vi "merFISH_move_to_XY_REF_position.vi"(5 "REF #":i32, 6 "Global parameters":T1 {"# repetitions" min=0; "Dt (s)" min=0 step=1; "Filter list" items=["ET665lp", "zet405/488/561/640m", "None", "None", "None", "None"]}, 7 "XY positions":dbl[][](array[numeric]), 8 "queue ASI stage":refnum<queue>, 10 "error in":errorcluster, 11 "REF positions":dbl[][](array[numeric])) -> (0 "Global parameters out":T1 {"# repetitions" min=0; "Dt (s)" min=0 step=1; "Filter list" items=["ET665lp", "zet405/488/561/640m", "None", "None", "None", "None"]}, 1 "error out":errorcluster, 3 "XY positions":dbl[][](array[numeric]))   [LabVIEW 2015]
uses:
  CONTROLS/Global parameters.ctl
  CONTROLS/Q_ASI_stage_element.ctl
  GLOBAL/Global_ASI_stage.vi
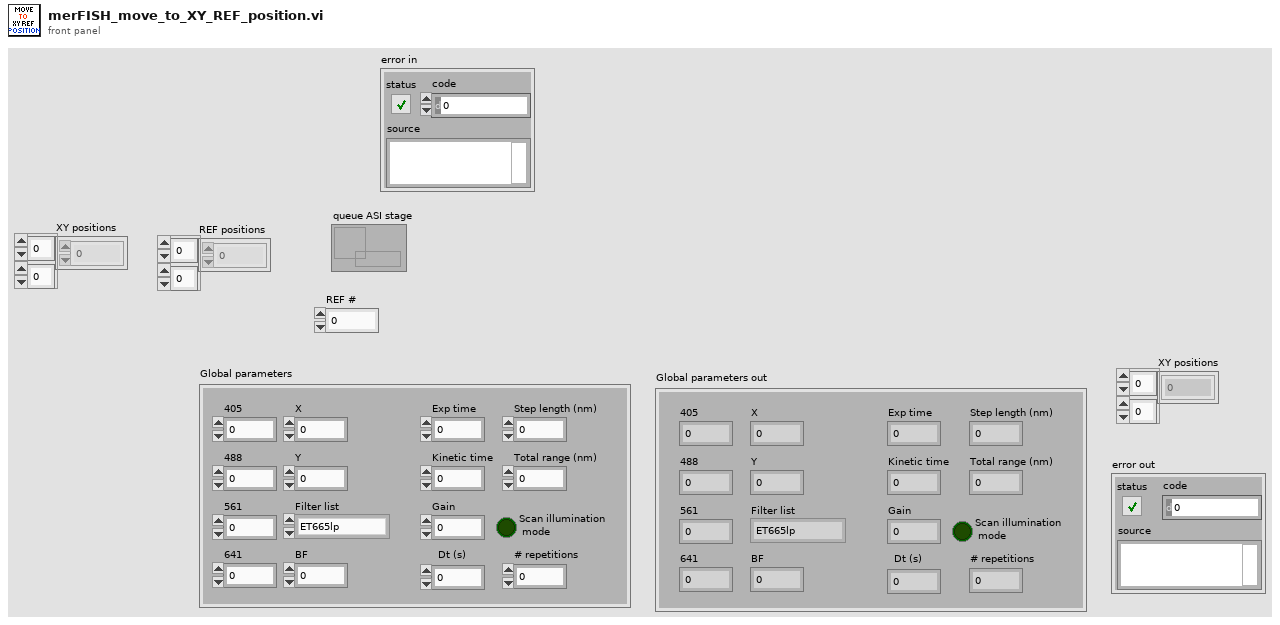
[diagram p1: front panel]
types:
  T1 = typedef "Global parameters.ctl" = cluster{"405":dbl, "488":dbl, "561":dbl, "641":dbl, "BF":dbl, "X":dbl, "Y":dbl, "Filter list":u16, "Exp time":sgl, "Kinetic time":sgl, "Gain":i32, "Step length (nm)":u32, "Total range (nm)":u32, "Scan illumination\n mode":bool, "Dt (s)":i32, "# repetitions":i32}
  T2 = typedef "Q_ASI_stage_element.ctl" = cluster{"variant":variant, "Instruction":enum16{"ASI_idle", "ASI_initialize", "ASI_error", "ASI_security_stop", "ASI_read_XYZ", "ASI_up", "ASI_down", "ASI_left", "ASI_right", "ASI_save_XY", "ASI_move_to_XY", "ASI_brightfield", "ASI_init_scan", "ASI_init_merFISH", "ASI_move_to_XY_merFISH", "ASI_move_to_Z_merFISH", "ASI_init_autofocus_search_merFISH", "ASI_close_autofocus_search_merFISH", "ASI_adjust_piezo_autofocus_merFISH", "ASI_set_piezo_autofocus_to_reference_position_merFISH_TL", "ASI_close_merFISH", "ASI_stop"}}
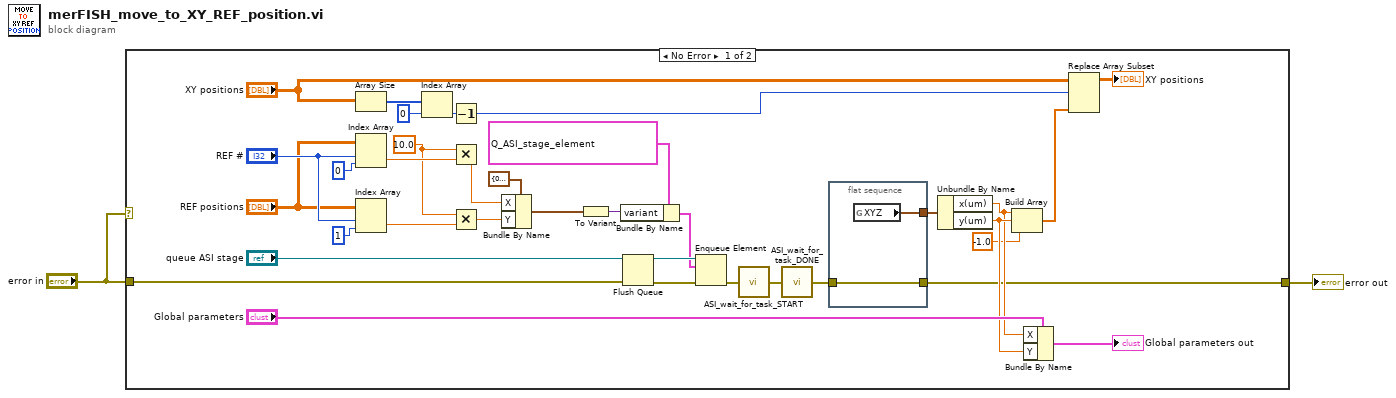
[diagram p0: block diagram]
diagram:
  n1 = case shown="No Error" "error in" {
    tunnel: "error in" -> [w26 w40]
    tunnel: [w7 w40] -> w2
    frame No Error {
      w28 = 10.0
      n2 = Array Size(array="XY positions") -> (size(s)=w36:i32[])
      n3 = Index Array(array="REF positions", index (row)="REF #", index (col)=0 ("disabled index (col)")) -> (element=w29:dbl)
      n4 = Index Array(array="REF positions", index (row)="REF #", index (col)=1 ("disabled index (col)")) -> (element=w30:dbl)
      n5 = Index Array(array=w36, index=0) -> (element=w34:i32)
      n6 = Decrement(x=w34) -> (x-1=w33:i32)
      n7 = Multiply(x=w28, y=w29) -> (x*y=w18:dbl)
      n8 = Multiply(x=w28, y=w30) -> (x*y=w17:dbl)
      n9 = Bundle By Name(cluster=cluster{"X":dbl, "Y":dbl} {"X"=0.0, "Y"=0.0} ("output cluster"), "X"=w18, "Y"=w17) -> (w5:cluster{"X":dbl, "Y":dbl})
      n10 = To Variant(anything=w5) -> (Variant=w22:variant)
      n11 = Bundle By Name(cluster=T2 {"variant"=variant, "Instruction"=enum."ASI_move_to_XY_merFISH"} ("Q_ASI_stage"), "variant"=w22) -> (w21:T2)
      n12 = Flush Queue(queue="queue ASI stage", error in (no error)=w26) -> (queue out=w24:refnum<queue>, error out=w25:errorcluster)  [unwired: 1 out]
      n13 = Enqueue Element(queue=w24, element=w21, error in (no error)=w25) -> (error out=w20:errorcluster)  [unwired: 1 in, 2 out]
      n14 = call "ASI_wait_for_task_START.vi"("error in"=w20) -> ("error out"=w19:errorcluster)
      n15 = call "ASI_wait_for_task_DONE.vi"("error in"=w19) -> ("error out"=w16:errorcluster)
      n16 = flat-sequence {
        tunnel: w16 -> [w39]
        tunnel: [w39] -> w7
        tunnel: [w38] -> w15
        frame #0 {
          n17 = global read "Global_ASI_stage.vi" "XYZ"() -> (w38:cluster{"x(um)":dbl, "y(um)":dbl, "z(um)":dbl})
        }
      }
      n18 = Unbundle By Name(w15) -> ("x(um)"=w12:dbl, "y(um)"=w13:dbl)
      n19 = Build Array(w12, w13, -1.0 ("element")) -> (w37:dbl[])
      n20 = Bundle By Name(cluster="Global parameters", "X"=w12, "Y"=w13) -> (→"Global parameters out":T1)
      n21 = Replace Array Subset(array="XY positions", new element=w37, index (row)=w33) -> (→"XY positions":dbl[][])  [unwired: 1 in]
    }
    frame Error {
    }
  }
  "error out" <- w2
